vi "get_data.vi"(9 "condition":string, 10 "table":string, 11 "columns":string[](array[string])) -> (0 "connection reference out":T1, 1 "Application Directory":path, 2 "connection information":path, 3 "Data":variant[][](array[variant]))   [LabVIEW 2014]
doc: "Used to get Data from Database table based on Table, Columns and condition (if any)"
uses:
  <vilib>/addons/database/Connection.llb/Conn ObjectReference.ctl
  <vilib>/addons/database/Connection.llb/DB Tools Open Connec (Path).vi
  <vilib>/addons/database/NI_Database_API.lvlib
panel:
  # "Used to get Data from Database table"
  # "Outputs"
  # "Inputs"
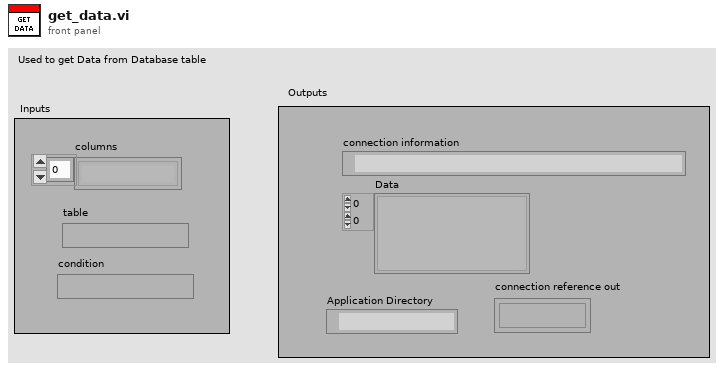
[diagram p1: front panel]
types:
  T1 = typedef "NI_Database_API.lvlib/Conn ObjectReference.ctl" = refnum<k1>
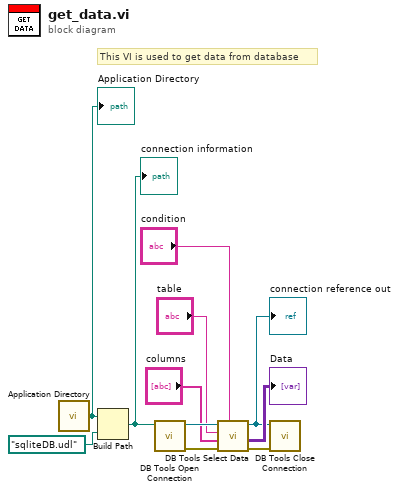
[diagram p0: block diagram]
diagram:
  # "This VI is used to get data from database"
  n1 = call <vilib>:"Application Directory.vi"() -> ("Application Directory"=w8:path)
  "Application Directory" <- w8
  n2 = Build Path(base path=w8, name or relative path=path "sqliteDB.udl" ("connection information")) -> (appended path=w7:path)
  "connection information" <- w7
  n3 = call-poly <vilib>:"DB Tools Open Connection.vi"("connection information"=w7) -> ("error out"=w10:errorcluster, "connection reference"=w11:T1)  [unwired: 7 in]
  n4 = call <vilib>:"DB Tools Select Data.vi"("condition"="condition", "error in (no error)"=w10, "columns"="columns", "table"="table", "connection reference"=w11) -> ("error out"=w1:errorcluster, "data"=→"Data":variant[][], "connection reference out"=w2:T1)  [unwired: 1 in]
  "connection reference out" <- w2
  n5 = call <vilib>:"DB Tools Close Connection.vi"("error in (no error)"=w1, "connection reference"=w2) -> ()  [unwired: 5 in, 1 out]
